vi "Special Query.vi"(5 "Termination Character (10)":u8=10, 7 "Enable Termination Character \n(Disable)":bool, 8 "error in (no error)":errorcluster, 9 "Timeout (10000ms)":u32=10000, 10 "Write Buffer":string, 11 "VISA resource name":refnum<visa-resource-name>) -> (0 "error out":errorcluster, 2 "Read Buffer":string, 3 "VISA resource name out":refnum<visa-resource-name>)   [LabVIEW 2009, in "DSO1K.lvlib"]
doc: "Writes the data and reads the returns the data ."
uses:
  <instrlib>/DSO1K/DSO1K.lvlib
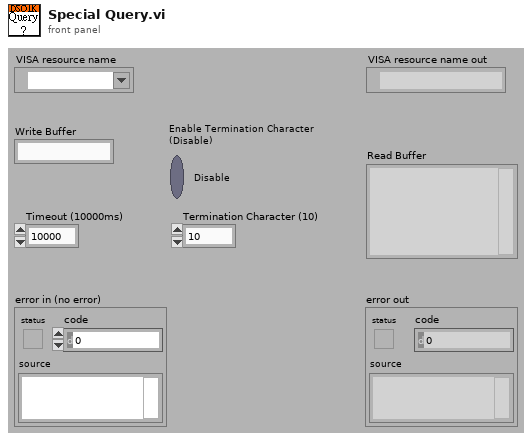
[diagram p1: front panel]
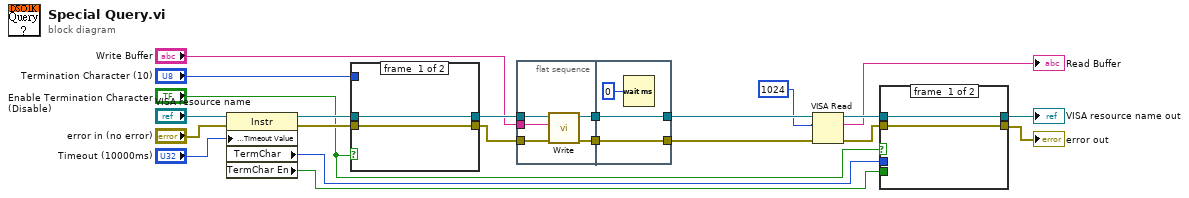
[diagram p0: block diagram]
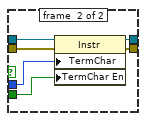
[diagram p2: hidden frame]
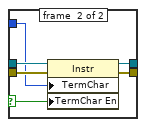
[diagram p3: hidden frame]
diagram:
  n1 = property class="Instr"(reference="VISA resource name", error in="error in (no error)", "General Settings:Timeout Value"="Timeout (10000ms)") -> (reference out=w19:refnum<visa-resource-name>, error out=w18:errorcluster, "TermChar"=w12:u8, "TermChar En"=w11:bool)
  n2 = case shown="True" "Enable Termination Character \n(Disable)" {
    selector: "Enable Termination Character \n(Disable)" -> [_ w26]
    tunnel: w19 -> [w24 w30]
    tunnel: w18 -> [w23 w29]
    tunnel: [w24 w28] -> w17
    tunnel: [w23 w27] -> w16
    tunnel: "Termination Character (10)" -> [_ w25]
    frame #0 {
    }
    frame #1 {
      n3 = property class="Instr"(reference=w30, error in=w29, "TermChar"=w25, "TermChar En"=w26) -> (reference out=w28:refnum<visa-resource-name>, error out=w27:errorcluster)
    }
  }
  n4 = flat-sequence {
    tunnel: w17 -> [w35]
    tunnel: w16 -> [w34]
    tunnel: "Write Buffer" -> [w33]
    tunnel: [w32] -> w10
    tunnel: [w31] -> w9
    tunnel: [w37] -> w4
    tunnel: [w38] -> w6
    tunnel: w10 -> [w38]
    tunnel: w9 -> [w37]
    frame #0 {
      n5 = call <instrlib>:"Write.vi"("error in (no error)"=w34, "Write Buffer (\"\")"=w33, "VISA resource name"=w35) -> ("error out"=w31:errorcluster, "VISA resource name out"=w32:refnum<visa-resource-name>)  [unwired: 6 in, 1 out]
    }
    frame #1 {
      n6 = Wait (ms)(milliseconds to wait=u32 0) -> ()  [unwired: 1 out]
    }
  }
  n7 = VISA Read(VISA resource name=w6, byte count=u32 1024, error in (no error)=w4) -> (VISA resource name out=w3:refnum<visa-resource-name>, read buffer=→"Read Buffer":string, error out=w1:errorcluster)  [unwired: 1 out]
  n8 = case shown="True" "Enable Termination Character \n(Disable)" {
    tunnel: w3 -> [w40 w46]
    tunnel: w1 -> [w39 w45]
    tunnel: [w40 w44] -> w13
    tunnel: [w39 w43] -> w14
    tunnel: w12 -> [_ w42]
    tunnel: w11 -> [_ w41]
    frame #0 {
    }
    frame #1 {
      n9 = property class="Instr"(reference=w46, error in=w45, "TermChar"=w42, "TermChar En"=w41) -> (reference out=w44:refnum<visa-resource-name>, error out=w43:errorcluster)
    }
  }
  "error out" <- w14
  "VISA resource name out" <- w13
